vi "LicenseBinding.vi"(7 "Library Directory":path, 8 "error in (no error)":errorcluster, 10 "product version":string, 11 "Package Display Name":string) -> (0 "error out":errorcluster, 3 "licensing successful?":bool)   [LabVIEW 2014]
uses:
  <vilib>/AddonLicensing/API.llb/_LV2P_ProductInformation.ctl
  <vilib>/AddonLicensing/API.llb/_LV2P_LicensingInformation.ctl
  <vilib>/AddonLicensing/API.llb/_LV2P_AuthorEncryptionInfo.ctl
  <vilib>/AddonLicensing/NI_LV2PLicAPI.lvlib
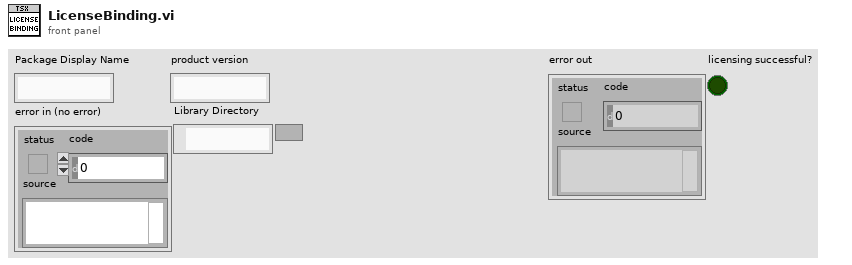
[diagram p1: front panel]
types:
  T1 = typedef "NI_LV2PLicAPI.lvlib/_LV2P_AuthorEncryptionInfo.ctl" = cluster{"encryption key id":string, "server key":string, "client key":string}
  T2 = enum8{"None", "Auto", "Web", "Auto | Web", "Phone", "Auto | Phone", "Web | Phone", "Auto | Web | Phone"}
  T3 = typedef "NI_LV2PLicAPI.lvlib/_LV2P_LicensingInformation.ctl" = cluster{"license file path":path, "license file password":string, "auto activation URL":string, "web activation URL":string, "phone activation number":string, "activation methods":enum8{"None", "Auto", "Web", "Auto | Web", "Phone", "Auto | Phone", "Web | Phone", "Auto | Web | Phone"}}
  T4 = typedef "NI_LV2PLicAPI.lvlib/_LV2P_ProductInformation.ctl" = cluster{"path to lvlib":path, "company name":string, "product name":string, "product version":string, "purchase page URL":string}
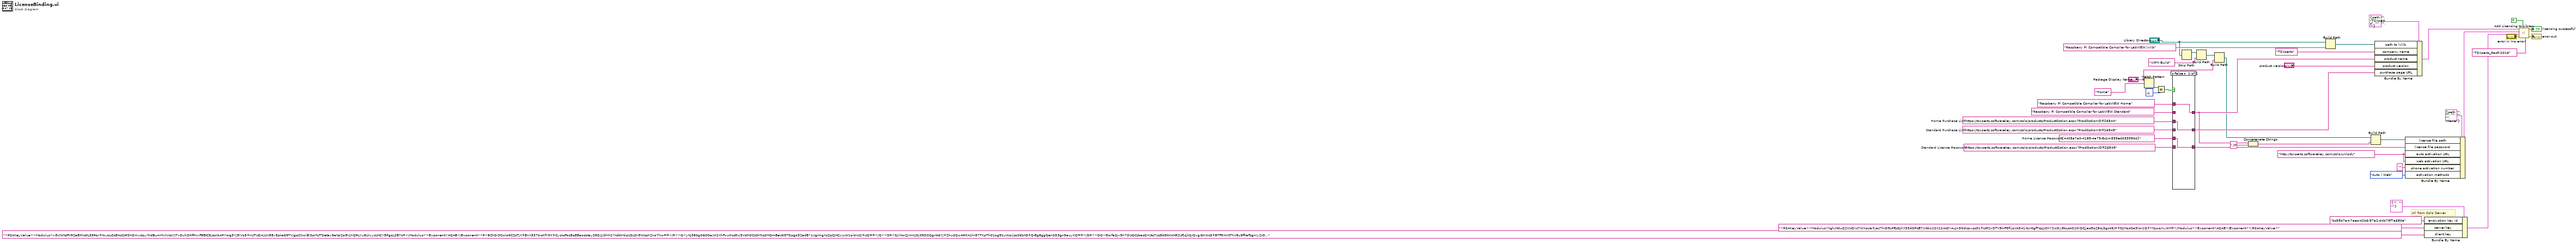
[diagram p0: block diagram]
diagram:
  w22 = "http://tsxperts.softwarekey.com/solo/unlock/" ("Standard License Password")
  w23 = "https://tsxperts.softwarekey.com/solo/products/ProductOption.aspx?ProdOptionID=26545"  # Standard License Password
  w25 = "{4405a7a0-4189-4a79-8c14-535ed033990d}"  # Home License Password
  w30 = "https://tsxperts.softwarekey.com/solo/products/ProductOption.aspx?ProdOptionID=26545"  # Standard Purchase Link
  w31 = "https://tsxperts.softwarekey.com/solo/products/ProductOption.aspx?ProdOptionID=26544"  # Home Purchase Link
  # "All from Solo Server"
  n1 = Match Pattern(string="Package Display Name", regular expression="Home") -> (offset past match=w38:i32)  [unwired: 1 in, 3 out]
  n2 = Equal?(x=w38, y=-1) -> (x = y?=w36:bool)
  n3 = case shown="False" w36 {
    tunnel: "Raspberry Pi Compatible Compiler for LabVIEW Home" ("regular expression") -> [w46 _]
    tunnel: "Raspberry Pi Compatible Compiler for LabVIEW Standard" ("regular expression") -> [_ w49]
    tunnel: [w46 w49] -> w20
    tunnel: w31 -> [w45 _]
    tunnel: w30 -> [_ w48]
    tunnel: [w45 w48] -> w29
    tunnel: w25 -> [w44 _]
    tunnel: [w44 w47] -> w24
    tunnel: w23 -> [_ w47]
    frame False {
    }
    frame True {
    }
  }
  n4 = Strip Path(path="Library Directory") -> (stripped path=w6:path)  [unwired: 1 out]
  n5 = Build Path(base path=w6, name or relative path="VIPM Build") -> (appended path=w3:path)
  n6 = Build Path(base path=w3, name or relative path="Package Display Name") -> (appended path=w1:path)
  n7 = Concatenate Strings(w20, ".lf" ("string")) -> (w18:string)
  n8 = Build Path(base path="Library Directory", name or relative path="Raspberry Pi Compatible Compiler for LabVIEW.lvlib") -> (appended path=w42:path)
  n9 = Build Path(base path=w1, name or relative path=w18) -> (appended path=w21:path)
  n10 = Bundle By Name(cluster=T4 {"path to lvlib"=path "", "company name"="TSXperts", "product name"="", "product version"="", "purchase page URL"=""} ("product information"), "path to lvlib"=w42, "company name"="TSXperts", "product name"=w20, "product version"="product version", "purchase page URL"=w29) -> (w40:T4)
  n11 = Bundle By Name(cluster=T3 {"license file path"=path "", "license file password"="", "auto activation URL"="", "web activation URL"="", "phone activation number"="", "activation methods"=enum."None"} ("licensing information"), "license file path"=w21, "license file password"=w24, "auto activation URL"=w22, "web activation URL"=w22, "phone activation number"="", "activation methods"=T2."Auto | Web") -> (w27:T3)
  n12 = Bundle By Name(cluster=T1 {"encryption key id"="", "server key"="", "client key"=""} ("author encryption information"), "encryption key id"="bc35b7a4-7aec-42b6-97a2-d4b79f7a680a", "server key"="<RSAKeyValue><Modulus>kgh/N0uQZVUQIis7WXqUa+jaz7hrD9LPEsSJKX33dOPcB7/nt0w1SX124c0YAuJn3OdUpvqs31+LtRZxDTV5krFGfijqVd34IjitLIr0gfTcpjJOKY2wDy8bLcAO10iQCjjasGqZ8Aj3gz45jH+OJMq4Sa3lzn1Q+YNLwqXv/4M=</Modulus><Exponent>AQAB</Exponent></RSAKeyValue>", "client key"="<RSAKeyValue><Modulus>vGr/WNsFVRZaEHkc0L39RoI+Nx/oLOsE4zCzPShDmvdpyiHdBumMvkVczYJTxDuhSHfPnvF8EtC3jssnb4PYArg3YJ9lVo5+nUTUDA/LkIG8v5pka69TV/gqCIkwiBiSpMUTDetax9aNpZoGVjKQRLYu8LkvyzUN2Y5PgqL2B7c=</Modulus><Exponent>AQAB</Exponent><P>8ChDi0CwloRCZsTJX+EnX337bisKfYRX+CyzAcFoz8qEEaocotayS9D/jjOhh2YkdbhNipUSLOiGWcqhZno7hw==</P><Q>yNj380gO60Oa/W2XhFxuHzc9V/3VcHDCzOMlqSMQmBeU03TDpgo3ZadEY1/rgnhgXsZqCJNCx/uW1oibVc2+UQ==</Q><DP>SJIiNwZJVnKJDj0RDSQgnb6YJ+ZhuSQw4RHA1hr37TKpTh01og92uWpijzoS6bN3+QrEg8ggQenSD3gn5auyKQ==</DP><DQ>GoifaSJx5h7OUQCzbacQXUtc7Uz5b5tWAN9ZUFjzjkQ/Qxg/6KWc3+8TF9XKNThV8u9ffraFsgnIyZrOeq1toQ==</DQ><InverseQ>ohRGgbvK6txzqb5jmb+CFQ8LCWfAuAxMvH3QSRtlhQk2/KEiNV3/WpSaaieZH1jFkRbvC8zv88odyOVxjvZXbA==</InverseQ><D>h/psN/MxAPw1mYfefONwYy9huSTEyY3/I/skj/F8AN2nsmIIApIQqcyjMglpbMhgGE2nQB0lHusUXfBNkJRFEksdB2SU7koVpZp28nJncAz6pJqMMssluOMldgBnQX7QmtHQhhKpAuIecTFBTd2ZklJNfKDuZ6/crv3hL41QdeE=</D></RSAKeyValue>") -> (w13:T1)
  n13 = call <vilib>:"Add Licensing to Library.vi"("new lvlib password"="T$Xperts_RasPi2016" ("current lvlib password"), "Enable Deactivation"=TRUE, "error in (no error)"="error in (no error)", "author encryption information"=w13, "licensing information"=w27, "product information"=w40) -> ("error out"=→"error out":errorcluster, "licensing successful?"=→"licensing successful?":bool)  [unwired: 4 in]
